vi "read TBM configuration.vi"(8 "error in":errorcluster, 11 "tag bus processing plugin editor node in":refnum<class "tag bus processing plugin editor node.lvclass">) -> (0 "error out":errorcluster, 2 "configuration":refnum<class "TBM configuration.lvclass">, 3 "tag bus processing plugin editor node out":refnum<class "tag bus processing plugin editor node.lvclass">)   [LabVIEW 2013, in "tag bus processing plugin editor node.lvclass"]
uses:
  tag bus processing plugin editor node.lvclass
  <vilib>/NI/Tag Bus Module Framework/root configuration/TBM configuration.lvclass
  tag bus processing plugin editor node.lvclass/tag bus processing plugin editor node.ctl
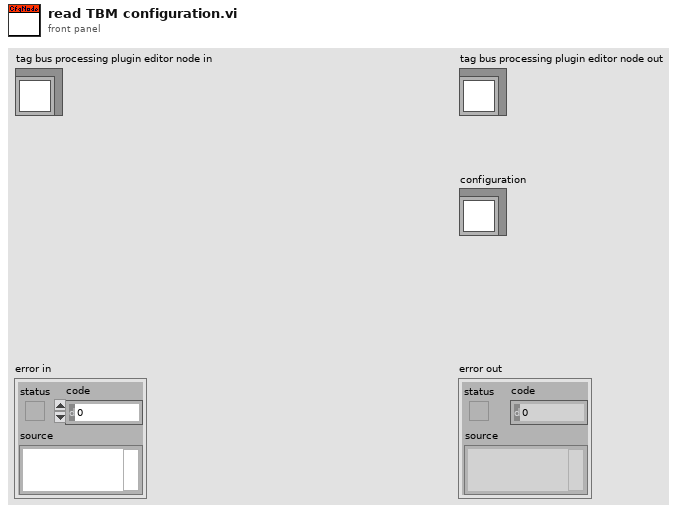
[diagram p1: front panel]
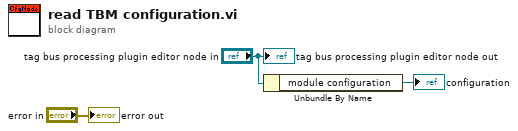
[diagram p0: block diagram]
diagram:
  n1 = Unbundle By Name("tag bus processing plugin editor node in") -> ("module configuration"=→"configuration":refnum<class "tag bus processing plugin module configuration.lvclass">)
  "error out" <- "error in"
  "tag bus processing plugin editor node out" <- "tag bus processing plugin editor node in"
